vi "ConvertSenseFormatElementsToItemList.vi"(11 "Sense Format Elements":T1[](array[typedef])=[enum."Current 1"]) -> (3 "Item List":string)   [LabVIEW 2012, in "Keithley-6482.lvlib"]
uses:
  Public/Controls/SenseFormatElement.ctl
  Keithley-6482.lvlib
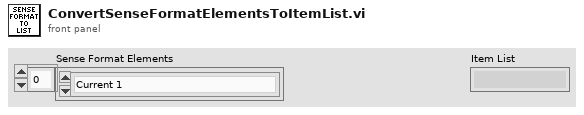
[diagram p1: front panel]
types:
  T1 = typedef "Keithley-6482.lvlib/SenseFormatElement.ctl" = enum16{"Current 1", "Current 2", "Time", "Status"}
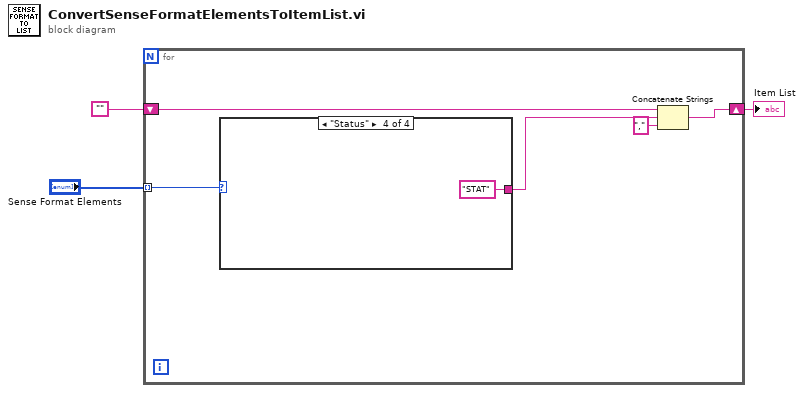
[diagram p0: block diagram]
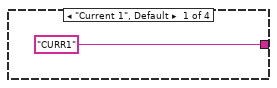
[diagram p2: hidden frame]
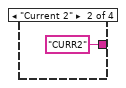
[diagram p3: hidden frame]
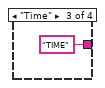
[diagram p4: hidden frame]
diagram:
  n1 = for {
    tunnel: "Sense Format Elements" -> [w6] mode=indexing
    shift-right: [w7] -> w1
    shift-left: "" -> [w8]
    n2 = case shown="\"Status\"" w6 {
      tunnel: ["CURR1" "CURR2" "TIME" "STAT"] -> w5
      frame "Current 1", Default {
      }
      frame "Current 2" {
      }
      frame "Time" {
      }
      frame "Status" {
      }
    }
    n3 = Concatenate Strings(w8, w5, "," ("string")) -> (w7:string)
  }
  "Item List" <- w1
